vi "Async Core.vi"(10 "Startup Promise":refnum<class "Promise.lvclass">, 11 "Module in":refnum<class "Module.lvclass">) -> ()   [LabVIEW 2020, in "Volatus.lvlib" / "Module.lvclass"]
uses:
  Module.lvclass
  lv-promises/Promises/Promise/Promise.lvclass
  State.ctl
  MessageQ Value/MessageQ Value.lvclass/MessageQ Value.ctl
  Module.lvclass/Module.ctl
  MessageQ Value/MessageQ Value.lvclass
  C:/dev/lv20CE/relink/lv-promises/Promises/Value/Value.lvclass
  MessageQ/MessageQ.lvclass
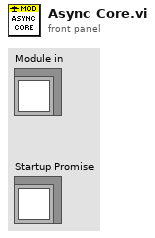
[diagram p1: front panel]
types:
  T1 = typedef "Volatus.lvlib/Module.lvclass/State.ctl" = enum16{"Unknown", "Launched", "Starting", "Running", "Stopping", "Stopped", "Error - Starting", "Error - Run", "Error - Stopping"}
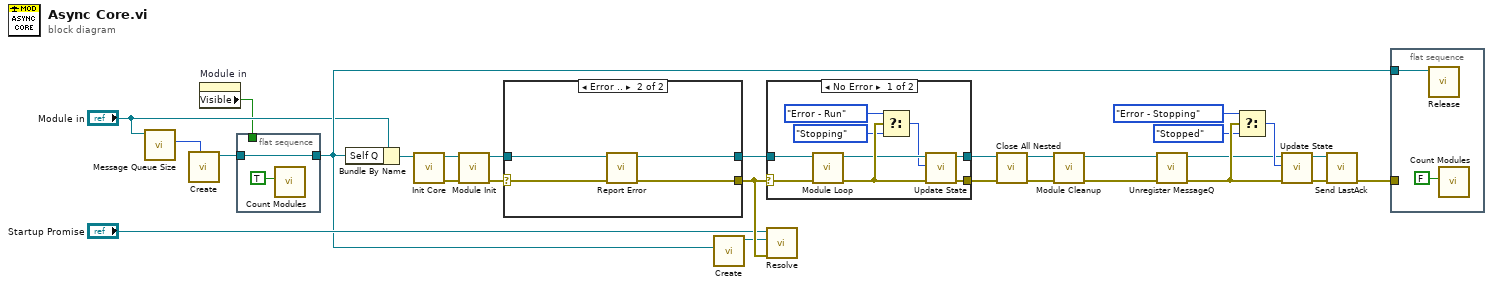
[diagram p0: block diagram]
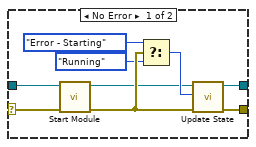
[diagram p2: hidden frame]
diagram:
  n1 = call-dynamic "Message Queue Size.vi"("Module in"="Module in") -> ("Queue Size (-1, Unlimited)"=w25:i32)  [unwired: 10 in]
  n2 = call "Create.vi"("Size (-1, Unlimited)"=w25) -> ("MessageQ out"=w26:refnum<class "MessageQ.lvclass">)  [unwired: 9 in, 1 out]
  n3 = property on="Module in" class="LVClassControl (strict)"() -> ("Visible"=w8:bool)  [unwired: 2 in, 2 out]
  n4 = flat-sequence {
    tunnel: w26 -> [w29]
    tunnel: [w29] -> w20
    tunnel: w8 -> [_]
    frame #0 {
      n5 = call "Count Modules.vi"("Increment"=TRUE) -> ()  [unwired: 11 in]
    }
  }
  n6 = Bundle By Name(cluster="Module in", "Self Q"=w20) -> (w12:refnum<class "Module.lvclass">)
  n7 = call "Init Core.vi"("Module in"=w12) -> ("error out"=w17:errorcluster, "Module out"=w21:refnum<class "Module.lvclass">)  [unwired: 9 in]
  n8 = call-dynamic "Module Init.vi"("error in (no error)"=w17, "Module in"=w21) -> ("error out"=w14:errorcluster, "Module out"=w15:refnum<class "Module.lvclass">)  [unwired: 8 in]
  n9 = case shown="Error .." w14 {
    selector: w14 -> [w37 w41]
    tunnel: w15 -> [w38 w43]
    tunnel: [w31 w40] -> w28
    tunnel: [w32 w42] -> w13
    frame No Error {
      n10 = call "Start Module.vi"("error in (no error)"=w37, "Module in"=w38) -> ("error out"=w39:errorcluster, "Module out"=w33:refnum<class "Module.lvclass">)  [unwired: 8 in]
      n11 = Select(t=State."Error - Starting" ("f"), s=w39, f=State."Running") -> (s? t:f=w34:T1)
      n12 = call "Update State.vi"("error in (no error)"=w39, "State"=w34, "Module in"=w33) -> ("error out"=w31:errorcluster, "Module out"=w32:refnum<class "Module.lvclass">)  [unwired: 7 in]
    }
    frame Error {
      n13 = call "Report Error.vi"("error in (no error)"=w41, "Module in"=w43) -> ("error out"=w40:errorcluster, "Module out"=w42:refnum<class "Module.lvclass">)  [unwired: 8 in]
    }
  }
  n14 = call "Create.vi"("MessageQ"=w20) -> ("MessageQ Value out"=w23:refnum<class "MessageQ Value.lvclass">)  [unwired: 10 in]
  n15 = case shown="No Error" w28 {
    selector: w28 -> [w44 w53]
    tunnel: w13 -> [w45 w54]
    tunnel: [w49 w54] -> w10
    tunnel: [w51 w53] -> w22
    frame No Error {
      n16 = call-dynamic "Module Loop.vi"("error in (no error)"=w44, "Module in"=w45) -> ("error out"=w52:errorcluster, "Module out"=w50:refnum<class "Module.lvclass">)  [unwired: 8 in]
      n17 = Select(t=State."Error - Run" ("State"), s=w52, f=State."Stopping") -> (s? t:f=w46:T1)
      n18 = call "Update State.vi"("error in (no error)"=w52, "State"=w46, "Module in"=w50) -> ("error out"=w51:errorcluster, "Module out"=w49:refnum<class "Module.lvclass">)  [unwired: 7 in]
    }
    frame Error {
    }
  }
  n19 = call "Resolve.vi"("error in (no error)"=w28, "Result"=w23, "Promise in"="Startup Promise") -> ()  [unwired: 7 in, 2 out]
  n20 = call "Close All Nested.vi"("error in (no error)"=w22, "Module in"=w10) -> ("error out"=w11:errorcluster, "Module out"=w9:refnum<class "Module.lvclass">)  [unwired: 8 in]
  n21 = call-dynamic "Module Cleanup.vi"("error in (no error)"=w11, "Module in"=w9) -> ("error out"=w27:errorcluster, "Module out"=w18:refnum<class "Module.lvclass">)  [unwired: 8 in]
  n22 = call "Unregister MessageQ.vi"("error in (no error)"=w27, "Module in"=w18) -> ("error out"=w7:errorcluster, "Module out"=w1:refnum<class "Module.lvclass">)  [unwired: 8 in]
  n23 = Select(t=State."Error - Stopping" ("State"), s=w7, f=State."Stopped") -> (s? t:f=w6:T1)
  n24 = call "Update State.vi"("error in (no error)"=w7, "State"=w6, "Module in"=w1) -> ("error out"=w3:errorcluster, "Module out"=w2:refnum<class "Module.lvclass">)  [unwired: 7 in]
  n25 = call "Send LastAck.vi"("error in (no error)"=w3, "Module in"=w2) -> ("error out"=w19:errorcluster)  [unwired: 9 in]
  n26 = flat-sequence {
    tunnel: w20 -> [w55]
    tunnel: w19 -> [_]
    frame #0 {
      n27 = call "Release.vi"("MessageQ in"=w55) -> ()  [unwired: 10 in, 1 out]
      n28 = call "Count Modules.vi"("Increment"=FALSE) -> ()  [unwired: 11 in]
    }
  }
